vi "SDO_Trajectory_BEGIN.vi"(11 "SWERVE_DRIVE_KINEMATICS":T1 {"SavedModuleStates"."Angle"."SIN" format="%13.4f"; "SavedModuleStates"."Angle"."COS" format="%13.4f"; "SavedModuleStates"."Angle"."VALUE" format="%13.4f"; "PrevCoR"."Y" format="%14.3f"; "PrevCoR"."X" format="%14.3f"; "Modules"."Y" format="%14.3f"; "Modules"."X" format="%14.3f"}) -> ()   [LabVIEW 2019]
uses:
  SDO_TRAJECTORY_GLOBALS.vi
  <vilib>/Analysis/Matrix/Datatypes/RealMatrix.ctl
  <vilib>/Analysis/Matrix/NI_Matrix.lvlib
  <vilib>/Rock Robotics/WPI/ThirdParty/JAS_Junk/TrajLib/TypeDef/TRANSLATION2D.ctl
  <vilib>/Rock Robotics/WPI/ThirdParty/JAS_Junk/TrajLib/Trajectory_Library.lvlib
  <vilib>/Rock Robotics/WPI/ThirdParty/JAS_Junk/TrajLib/TypeDef/ROTATION2D.ctl
  <vilib>/Rock Robotics/WPI/ThirdParty/JAS_Junk/TrajLib/TypeDef/SWERVE_DRIVE_MODULE_STATE.ctl
  <vilib>/Rock Robotics/WPI/ThirdParty/JAS_Junk/TrajLib/TypeDef/SWERVE_DRIVE_KINEMATICS.ctl
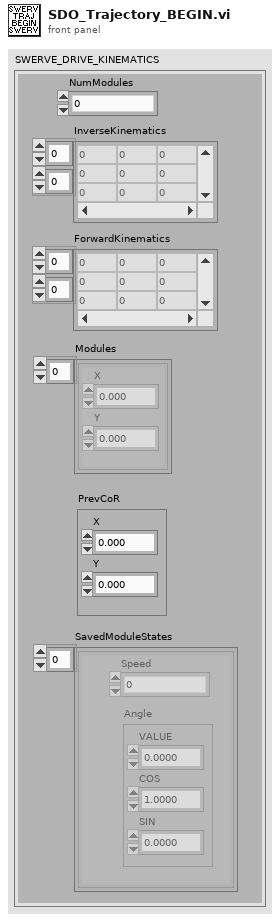
[diagram p1: front panel]
types:
  T1 = typedef "Trajectory_Library.lvlib/SWERVE_DRIVE_KINEMATICS.ctl" = cluster{"NumModules":i32, "InverseKinematics":T2, "ForwardKinematics":T2, "Modules":T3[], "PrevCoR":T3, "SavedModuleStates":T4[]}
  T2 = typedef "NI_Matrix.lvlib/RealMatrix.ctl" = dbl[][]
  T3 = typedef "Trajectory_Library.lvlib/TRANSLATION2D.ctl" = cluster{"X":dbl, "Y":dbl}
  T4 = typedef "Trajectory_Library.lvlib/SWERVE_DRIVE_MODULE_STATE.ctl" = cluster{"Speed":dbl, "Angle":T5}
  T5 = typedef "Trajectory_Library.lvlib/ROTATION2D.ctl" = cluster{"VALUE":dbl, "COS":dbl, "SIN":dbl}
  T6 = typedef "Trajectory_Library.lvlib/TRAJECTORY.ctl" = cluster{"TotalTImeSecs":dbl, "States":T7[]}
  T7 = typedef "Trajectory_Library.lvlib/TRAJ_STATE.ctl" = cluster{"TimeSeconds":dbl, "Velocity":dbl, "Acceleration":dbl, "POSE":T8, "Curvature":dbl}
  T8 = typedef "Trajectory_Library.lvlib/POSE2D.ctl" = cluster{"TRANSLATION":T3, "ROTATION":T5}
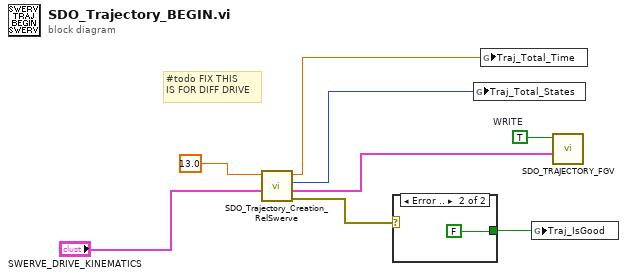
[diagram p0: block diagram]
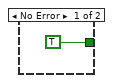
[diagram p2: hidden frame]
diagram:
  w7 = TRUE  # WRITE
  # "#todo FIX THIS\nIS FOR DIFF DRIVE"
  n1 = call "SDO_Trajectory_Creation_RelSwerve.vi"("SWERVE_DRIVE_KINEMATICS"="SWERVE_DRIVE_KINEMATICS", "Max Velocity Ft/Sec"=13.0) -> ("Trajectory  creation error"=w5:errorcluster, "Relative Trajectory"=w6:T6, "Trajectory Items"=w3:i32, "TotalTImeSecs"=w4:dbl)  [unwired: 6 in]
  n2 = case shown="Error .." w5 {
    tunnel: [TRUE FALSE] -> w8
    frame No Error {
    }
    frame Error {
    }
  }
  n3 = global write "SDO_TRAJECTORY_GLOBALS.vi" "Traj_Total_States"(w3) -> ()
  n4 = global write "SDO_TRAJECTORY_GLOBALS.vi" "Traj_Total_Time"(w4) -> ()
  n5 = global write "SDO_TRAJECTORY_GLOBALS.vi" "Traj_IsGood"(w8) -> ()
  n6 = call "SDO_TRAJECTORY_FGV.vi"("inTRAJECTORY"=w6, "WRITE"=w7) -> ()  [unwired: 9 in, 1 out]
